vi "WLAN - TV - RW - ReadTestVectorFile(Rx).vi"() -> (4 "PER Sweep Settings(Wfm * FreQ * Pwr)":T2[][][](array[typedef])=[[[{"Wfm_Index"=0, "Power Level Settings"={"Stop Power Level(dBm)"=-87.0, "Start Power Level(dBm)"=-67.0, "Step Size"=1.0}, "Carrier Frequency(Hz)"=2412000000.0, "# Freq Points"=4}], [{"Wfm_Index"=0, "Power Level Settings"={"Stop Power Level(dBm)"=-87.0, "Start Power Level(dBm)"=-67.0, "Step Size"=1.0}, "Carrier Frequency(Hz)"=5180000000.0, "# Freq Points"=4}], [{"Wfm_Index"=0, "Power Level Settings"={"Stop Power Level(dBm)"=-87.0, "Start Power Level(dBm)"=-67.0, "Step Size"=1.0}, "Carrier Frequency(Hz)"=5500000000.0, "# Freq Points"=4}], [{"Wfm_Index"=0, "Power Level Settings"={"Stop Power Level(dBm)"=-87.0, "Start Power Level(dBm)"=-67.0, "Step Size"=1.0}, "Carrier Frequency(Hz)"=5700000000.0, "# Freq Points"=4}]], [[{"Wfm_Index"=1, "Power Level Settings"={"Stop Power Level(dBm)"=-75.0, "Start Power Level(dBm)"=-55.0, "Step Size"=1.0}, "Carrier Frequency(Hz)"=2412000000.0, "# Freq Points"=4}], [{"Wfm_Index"=1, "Power Level Settings"={"Stop Power Level(dBm)"=-75.0, "Start Power Level(dBm)"=-55.0, "Step Size"=1.0}, "Carrier Frequency(Hz)"=5180000000.0, "# Freq Points"=4}], [{"Wfm_Index"=1, "Power Level Settings"={"Stop Power Level(dBm)"=-75.0, "Start Power Level(dBm)"=-55.0, "Step Size"=1.0}, "Carrier Frequency(Hz)"=5500000000.0, "# Freq Points"=4}], [{"Wfm_Index"=1, "Power Level Settings"={"Stop Power Level(dBm)"=-75.0, "Start Power Level(dBm)"=-55.0, "Step Size"=1.0}, "Carrier Frequency(Hz)"=5700000000.0, "# Freq Points"=4}]], [[{"Wfm_Index"=2, "Power Level Settings"={"Stop Power Level(dBm)"=-80.0, "Start Power Level(dBm)"=-60.0, "Step Size"=1.0}, "Carrier Frequency(Hz)"=2412000000.0, "# Freq Points"=4}], [{"Wfm_Index"=2, "Power Level Settings"={"Stop Power Level(dBm)"=-80.0, "Start Power Level(dBm)"=-60.0, "Step Size"=1.0}, "Carrier Frequency(Hz)"=5180000000.0, "# Freq Points"=4}], [{"Wfm_Index"=2, "Power Level Settings"={"Stop Power Level(dBm)"=-80.0, "Start Power Level(dBm)"=-60.0, "Step Size"=1.0}, "Carrier Frequency(Hz)"=5500000000.0, "# Freq Points"=4}], [{"Wfm_Index"=2, "Power Level Settings"={"Stop Power Level(dBm)"=-80.0, "Start Power Level(dBm)"=-60.0, "Step Size"=1.0}, "Carrier Frequency(Hz)"=5700000000.0, "# Freq Points"=4}]], [[{"Wfm_Index"=3, "Power Level Settings"={"Stop Power Level(dBm)"=-75.0, "Start Power Level(dBm)"=-55.0, "Step Size"=1.0}, "Carrier Frequency(Hz)"=2412000000.0, "# Freq Points"=4}], [{"Wfm_Index"=3, "Power Level Settings"={"Stop Power Level(dBm)"=-75.0, "Start Power Level(dBm)"=-55.0, "Step Size"=1.0}, "Carrier Frequency(Hz)"=5180000000.0, "# Freq Points"=4}], [{"Wfm_Index"=3, "Power Level Settings"={"Stop Power Level(dBm)"=-75.0, "Start Power Level(dBm)"=-55.0, "Step Size"=1.0}, "Carrier Frequency(Hz)"=5500000000.0, "# Freq Points"=4}], [{"Wfm_Index"=3, "Power Level Settings"={"Stop Power Level(dBm)"=-75.0, "Start Power Level(dBm)"=-55.0, "Step Size"=1.0}, "Carrier Frequency(Hz)"=5700000000.0, "# Freq Points"=4}]]], 6 "Waveform Generation Settings":T1[](array[typedef])=[{"Standard"=0, "Channel Bandwidth (Hz)"=20000000.0, "Idle Interval (s)"=0.0001, "MCS Index"=0, "80211n PLCP Frame Format"=0, "Payload Data Length (bytes)"=600, "OFDM Data Rate (Mbps)"=3, "DSSS Data Rate (Mbps)"=0, "Wfm_Index"=0}, {"Standard"=0, "Channel Bandwidth (Hz)"=20000000.0, "Idle Interval (s)"=0.0001, "MCS Index"=0, "80211n PLCP Frame Format"=0, "Payload Data Length (bytes)"=700, "OFDM Data Rate (Mbps)"=7, "DSSS Data Rate (Mbps)"=0, "Wfm_Index"=1}, {"Standard"=3, "Channel Bandwidth (Hz)"=20000000.0, "Idle Interval (s)"=0.0001, "MCS Index"=4, "80211n PLCP Frame Format"=0, "Payload Data Length (bytes)"=700, "OFDM Data Rate (Mbps)"=0, "DSSS Data Rate (Mbps)"=0, "Wfm_Index"=2}, {"Standard"=3, "Channel Bandwidth (Hz)"=20000000.0, "Idle Interval (s)"=0.0001, "MCS Index"=7, "80211n PLCP Frame Format"=0, "Payload Data Length (bytes)"=700, "OFDM Data Rate (Mbps)"=0, "DSSS Data Rate (Mbps)"=0, "Wfm_Index"=3}] {"DSSS Data Rate (Mbps)" items=["1", "2", "5.5 CCK", "5.5 PBCC", "11 CCK", "11 PBCC", "22", "33"]; "OFDM Data Rate (Mbps)" items=["6", "9", "12", "18", "24", "36", "48", "54"]; "80211n PLCP Frame Format" items=["Mixed Format", "Greenfield Format"]; "Standard" items=["80211A/G/J/P OFDM", "80211B/G DSSS", "80211G DSSSOFDM", "80211N MIMOOFDM", "80211AC MIMOOFDM"]}, 8 "#Packets":i32=100, 10 "PER Threshold":i32=10)   [LabVIEW 2011]
uses:
  Includes/WLAN - TV - RW - INC - Rx_PER_Sweep_Settings.ctl
  Includes/WLAN - TV - RW - INC - Rx_PER_Wfm_Settings.ctl
  <vilib>/Utility/file.llb/Read From Spreadsheet File (string).vi
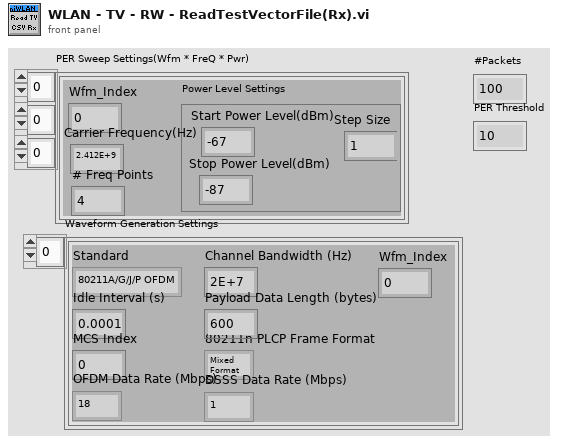
[diagram p1: front panel]
types:
  T1 = typedef "WLAN - TV - RW - INC - Rx_PER_Wfm_Settings.ctl" = cluster{"Standard":i32, "Channel Bandwidth (Hz)":dbl, "Idle Interval (s)":dbl, "MCS Index":i32, "80211n PLCP Frame Format":i32, "Payload Data Length (bytes)":i32, "OFDM Data Rate (Mbps)":i32, "DSSS Data Rate (Mbps)":i32, "Wfm_Index":i32}
  T2 = typedef "WLAN - TV - RW - INC - Rx_PER_Sweep_Settings.ctl" = cluster{"Wfm_Index":i32, "Power Level Settings":cluster{"Stop Power Level(dBm)":dbl, "Start Power Level(dBm)":dbl, "Step Size":dbl}, "Carrier Frequency(Hz)":dbl, "# Freq Points":i32}
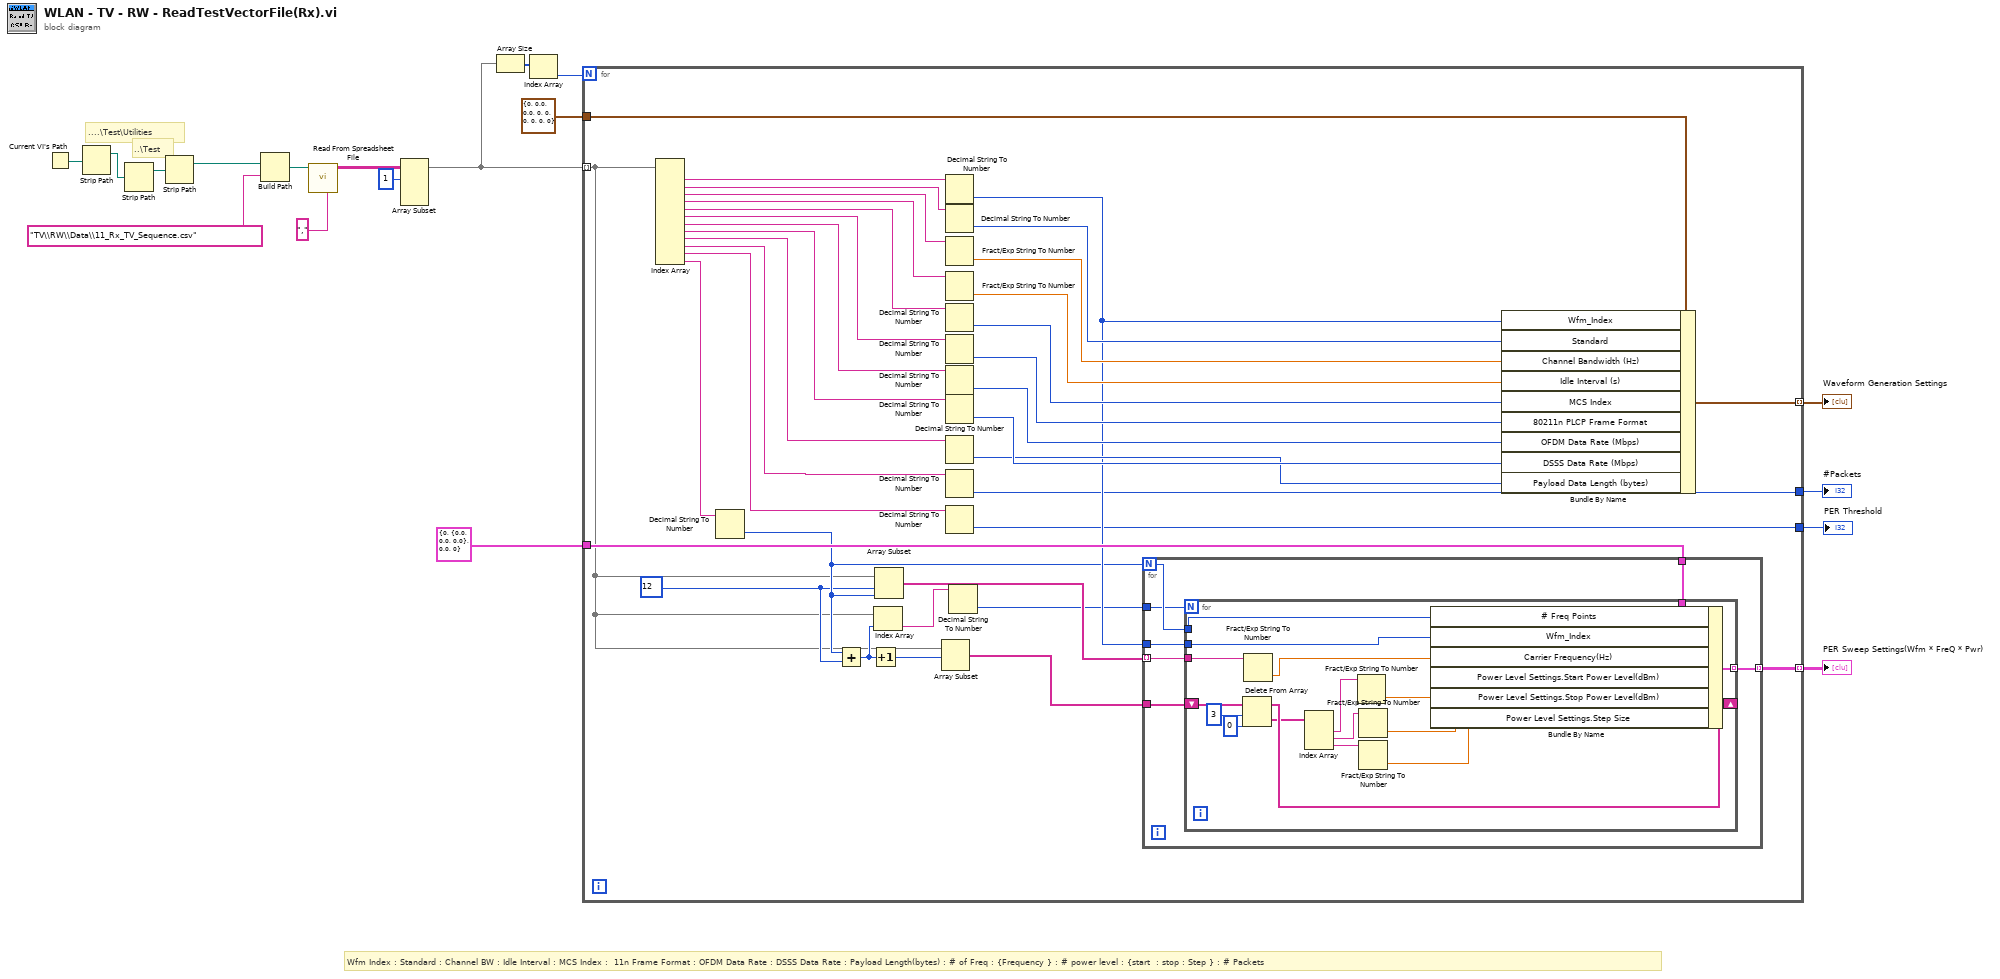
[diagram p0: block diagram]
diagram:
  # "....\\Test\\Utilities"
  # "..\\Test"
  # "Wfm Index : Standard : Channel BW : Idle Interval : MCS Index :  11n Frame Format : OFDM Data Rate : DSSS Data Rate : Payload Length(bytes) : # of Freq : {Frequency } : # power level : {start  : stop : Step } : # Packets"
  n1 = Current VI's Path() -> (path=w2:path)
  n2 = Strip Path(path=w2) -> (stripped path=w3:path)  [unwired: 1 out]
  n3 = Strip Path(path=w3) -> (stripped path=w4:path)  [unwired: 1 out]
  n4 = Strip Path(path=w4) -> (stripped path=w6:path)  [unwired: 1 out]
  n5 = Build Path(base path=w6, name or relative path="TV\\RW\\Data\\11_Rx_TV_Sequence.csv") -> (appended path=w10:path)
  n6 = call-poly <vilib>:"Read From Spreadsheet File.vi"("delimiter (\\t)"="," ("delimiter (\\t)"), "file path (dialog if empty)"=w10) -> ("all rows"=w8:string[][])  [unwired: 5 in, 4 out]
  n7 = Array Subset(array=w8, index (row)=1 ("index")) -> (w9:string[][])  [unwired: 3 in]
  n8 = Array Size(array=w9) -> (size(s)=w17:i32[])
  n9 = Index Array(array=w17) -> (element=w16:i32)  [unwired: 1 in]
  n10 = for {
    N: w16 -> [_]
    tunnel: w9 -> [w24] mode=indexing
    tunnel: T2 {"Wfm_Index"=0, "Power Level Settings"={"Stop Power Level(dBm)"=0.0, "Start Power Level(dBm)"=0.0, "Step Size"=0.0}, "Carrier Frequency(Hz)"=0.0, "# Freq Points"=0} ("Sweep Settings") -> [w35]
    tunnel: T1 {"Standard"=0, "Channel Bandwidth (Hz)"=0.0, "Idle Interval (s)"=0.0, "MCS Index"=0, "80211n PLCP Frame Format"=0, "Payload Data Length (bytes)"=0, "OFDM Data Rate (Mbps)"=0, "DSSS Data Rate (Mbps)"=0, "Wfm_Index"=0} ("Rx Measurements Settings") -> [w53]
    tunnel: [w36] -> w13 mode=indexing
    tunnel: [w34] -> w12 mode=indexing
    tunnel: [w22] -> w11
    tunnel: [w19] -> w1
    w30 = 12 ("index")
    n11 = Index Array(array=w24) -> (element #1=w54:string, element #2=w52:string, element #3=w51:string, element #4=w50:string, element #5=w49:string, element #6=w48:string, element #7=w47:string, element #8=w46:string, element #9=w45:string, element #10=w23:string, element #11=w20:string, element #12=w21:string)  [unwired: 12 in]
    n12 = Decimal String To Number(string=w21) -> (number=w31:i32)  [unwired: 2 in, 1 out]
    n13 = Add(x=w31, y=w30) -> (x+y=w29:i32)
    n14 = Increment(x=w29) -> (x+1=w25:i32)
    n15 = Index Array(array=w24, index=w29) -> (element=w28:string)
    n16 = Array Subset(array=w24, index=w30, length=w31) -> (w33:string[])
    n17 = Array Subset(array=w24, index=w25) -> (w27:string[])  [unwired: 1 in]
    n18 = Decimal String To Number(string=w54) -> (number=w32:i32)  [unwired: 2 in, 1 out]
    n19 = Decimal String To Number(string=w52) -> (number=w44:i32)  [unwired: 2 in, 1 out]
    n20 = Fract/Exp String To Number(string=w51) -> (number=w43:dbl)  [unwired: 3 in, 1 out]
    n21 = Fract/Exp String To Number(string=w50) -> (number=w42:dbl)  [unwired: 3 in, 1 out]
    n22 = Decimal String To Number(string=w49) -> (number=w41:i32)  [unwired: 2 in, 1 out]
    n23 = Decimal String To Number(string=w48) -> (number=w40:i32)  [unwired: 2 in, 1 out]
    n24 = Decimal String To Number(string=w47) -> (number=w39:i32)  [unwired: 2 in, 1 out]
    n25 = Decimal String To Number(string=w46) -> (number=w38:i32)  [unwired: 2 in, 1 out]
    n26 = Decimal String To Number(string=w45) -> (number=w37:i32)  [unwired: 2 in, 1 out]
    n27 = Decimal String To Number(string=w23) -> (number=w22:i32)  [unwired: 2 in, 1 out]
    n28 = Decimal String To Number(string=w20) -> (number=w19:i32)  [unwired: 2 in, 1 out]
    n29 = Decimal String To Number(string=w28) -> (number=w26:i32)  [unwired: 2 in, 1 out]
    n30 = for {
      N: w31 -> [w57]
      tunnel: w33 -> [w61] mode=indexing
      tunnel: w32 -> [w60]
      tunnel: w35 -> [w59]
      tunnel: [w58] -> w34 mode=indexing
      tunnel: w26 -> [w56]
      tunnel: w27 -> [w55]
      n31 = for {
        N: w56 -> [_]
        tunnel: w61 -> [w74]
        tunnel: w60 -> [w77]
        tunnel: w59 -> [w78]
        tunnel: [w76] -> w58 mode=indexing
        tunnel: w57 -> [w75]
        shift-right: [w69] -> _
        shift-left: w55 -> [w72]
        n32 = Delete From Array(array=w72, length=3, index=0) -> (deleted portion=w68:string[], array with subset deleted=w69:string[])
        n33 = Fract/Exp String To Number(string=w74) -> (number=w73:dbl)  [unwired: 3 in, 1 out]
        n34 = Index Array(array=w68) -> (element #1=w67:string, element #2=w66:string, element #3=w65:string)  [unwired: 3 in]
        n35 = Fract/Exp String To Number(string=w67) -> (number=w62:dbl)  [unwired: 3 in, 1 out]
        n36 = Fract/Exp String To Number(string=w66) -> (number=w63:dbl)  [unwired: 3 in, 1 out]
        n37 = Fract/Exp String To Number(string=w65) -> (number=w64:dbl)  [unwired: 3 in, 1 out]
        n38 = Bundle By Name(cluster=w78, "# Freq Points"=w75, "Wfm_Index"=w77, "Carrier Frequency(Hz)"=w73, "Power Level Settings.Start Power Level(dBm)"=w62, "Power Level Settings.Stop Power Level(dBm)"=w63, "Power Level Settings.Step Size"=w64) -> (w76:T2)
      }
    }
    n39 = Bundle By Name(cluster=w53, "Wfm_Index"=w32, "Standard"=w44, "Channel Bandwidth (Hz)"=w43, "Idle Interval (s)"=w42, "MCS Index"=w41, "80211n PLCP Frame Format"=w40, "OFDM Data Rate (Mbps)"=w39, "DSSS Data Rate (Mbps)"=w38, "Payload Data Length (bytes)"=w37) -> (w36:T1)
  }
  "PER Sweep Settings(Wfm * FreQ * Pwr)" <- w12
  "Waveform Generation Settings" <- w13
  "#Packets" <- w11
  "PER Threshold" <- w1
